vi "OA Get Int.vi"(9 "iIntValue":i32, 10 "pcModeParam":string, 11 "pcModeName":string) -> (1 "iIntValue out":i32, 3 "function return":u32)   [LabVIEW 2018, in "Copy of Andor SDK.lvlib"]
doc: "EXPNETTYPE unsigned int WINAPI OA_GetInt(const char * const pcModeName, const char * const pcModeParam, int * iIntValue);"
uses:
  Copy of Andor SDK.lvlib
  <userlib>/Andor SDK/ATMCD32D.dll
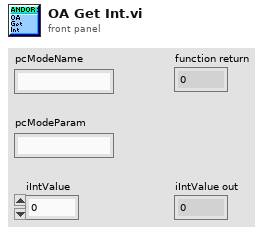
[diagram p1: front panel]
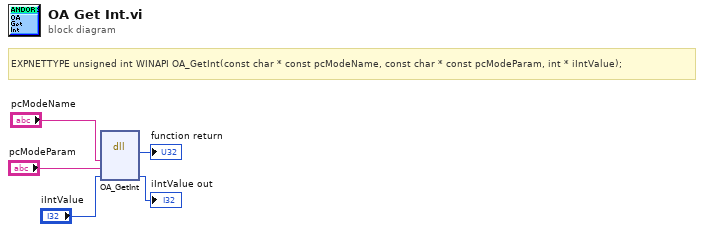
[diagram p0: block diagram]
diagram:
  # "EXPNETTYPE unsigned int WINAPI OA_GetInt(const char * const pcModeName, const char * const pcModeParam, int * iIntValue);"
  n1 = dll-call lib="C:/Program Files (x86)/National Instruments/LabVIEW 2018/user.lib/Andor SDK/ATMCD32D.*" fn="OA_GetInt"("pcModeName"="pcModeName", "pcModeParam"="pcModeParam", "iIntValue"="iIntValue") -> (→"function return":u32, "iIntValue"=→"iIntValue out":i32)  [unwired: 5 in, 2 out]
